vi "LINC Create Telemetry Definition.vi"(8 "error in (no error)":errorcluster, 10 "path":path, 11 "LINC session":refnum<class "LINC.lvclass">) -> (0 "error out":errorcluster, 3 "dup LINC session":refnum<class "LINC.lvclass">)   [LabVIEW 2018, in "STEPkgDriver_LINC.lvlib" / "LINC.lvclass"]
uses:
  LINC.lvclass
  STEPkgDriver_LINC.lvlib
  LINC Global Mode.ctl
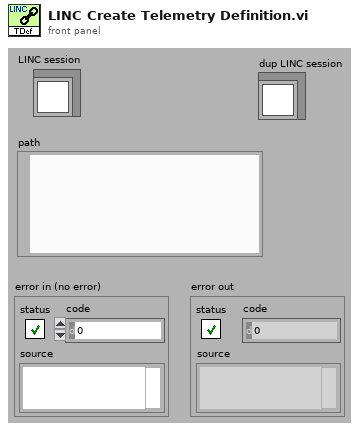
[diagram p1: front panel]
types:
  T1 = typedef "STEPkgDriver_LINC.lvlib/LINC Global Mode.ctl" = enum16{"INIT", "CLEAR", "ADD_PKT_HDR", "ADD_PKT", "GET_PKT_NAMES", "GET_PKT_DESC", "GET_PKT_HDR", "GET_PKT", "SET_PKT", "SET_DATA", "SIM_EN", "SIM_DS"}
  T2 = typedef "STEPkgDriver_LINC.lvlib/LINC Format Prototype.ctl" = cluster{"type":string, "bit offset":i32, "bit size":i32, "format":string, "unit":string, "description":string, "state values":i64[], "states":string[], "max":string, "min":string, "default":string, "array":bool, "bit element size":i32, "poly bound":dbl[], "poly scale":cluster{"coefficients":dbl[]}[], "labview size":i32, "simulate":bool, "ID":bool, "required":bool}
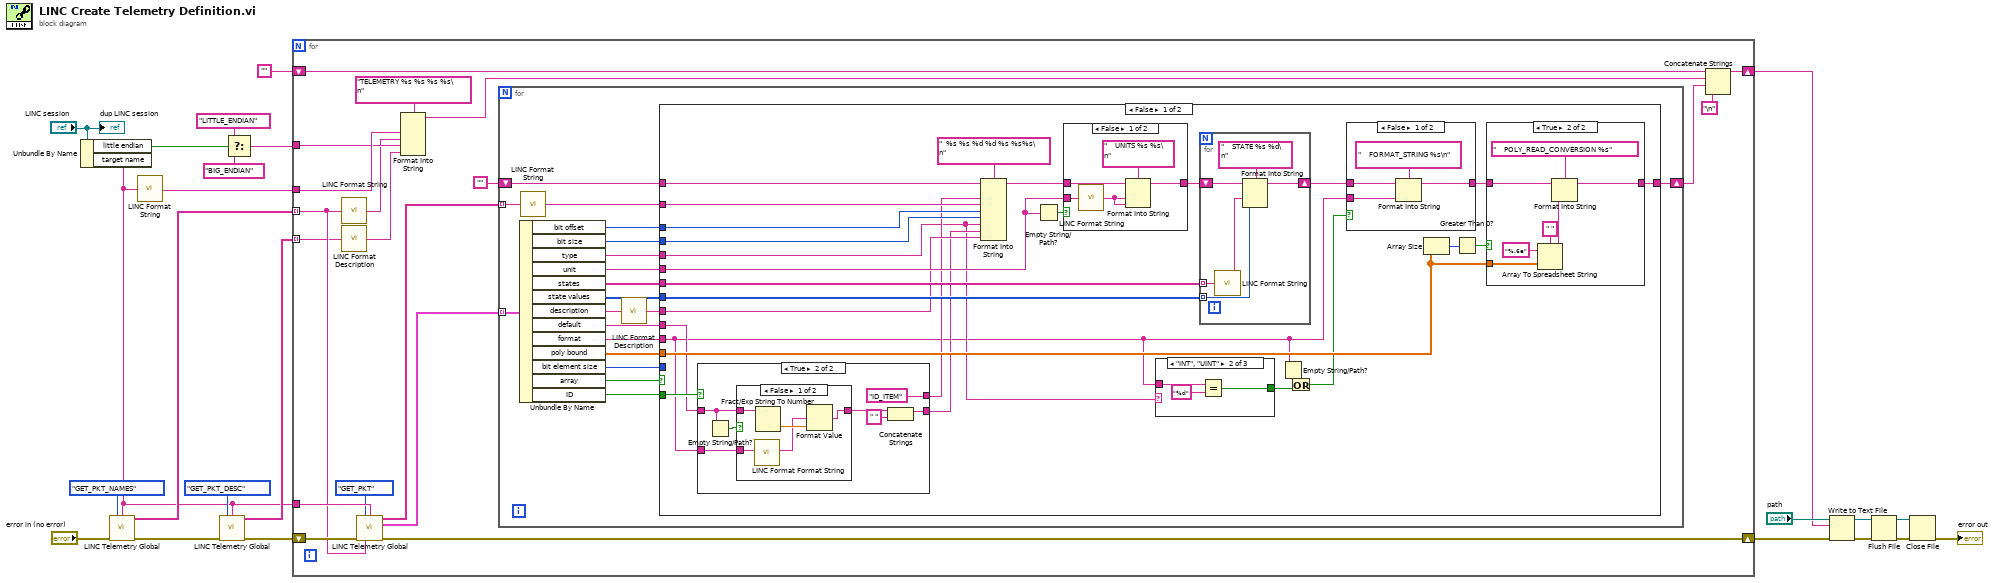
[diagram p0: block diagram]
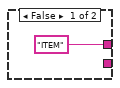
[diagram p2: hidden frame]
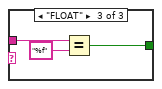
[diagram p5: hidden frame]
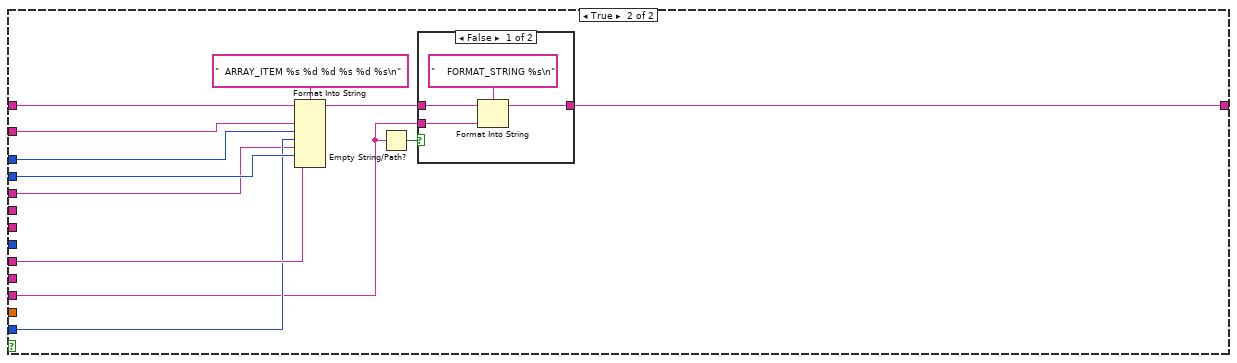
[diagram p9: hidden frame]
diagram:
  n1 = Unbundle By Name("LINC session") -> ("little endian"=w4:bool, "target name"=w1:string)
  n2 = call "LINC Telemetry Global.vi"("mode"=LINC_Global_Mode."GET_PKT_NAMES", "target name"=w1, "error in (no error)"="error in (no error)") -> ("values out"=w11:string[], "error out"=w15:errorcluster)  [unwired: 8 in, 3 out]
  n3 = call "LINC Format String.vi"("string in"=w1) -> ("string out"=w2:string)
  n4 = call "LINC Telemetry Global.vi"("mode"=LINC_Global_Mode."GET_PKT_DESC", "target name"=w1, "error in (no error)"=w15) -> ("values out"=w10:string[], "error out"=w14:errorcluster)  [unwired: 8 in, 3 out]
  n5 = Select(t="LITTLE_ENDIAN", s=w4, f="BIG_ENDIAN") -> (s? t:f=w3:string)
  n6 = for {
    tunnel: w2 -> [w42]
    shift-right: [w38] -> w16
    shift-left: "" -> [w39]
    shift-right: [w35] -> w12
    shift-left: w14 -> [w36]
    tunnel: w11 -> [w27] mode=indexing
    tunnel: w10 -> [w25] mode=indexing
    tunnel: w1 -> [w34]
    tunnel: w3 -> [w28]
    n7 = call "LINC Format String.vi"("string in"=w27) -> ("string out"=w26:string)
    n8 = call "LINC Format Description.vi"("string in"=w25) -> ("string out"=w24:string)
    n9 = call "LINC Telemetry Global.vi"("mode"=LINC_Global_Mode."GET_PKT", "target name"=w34, "error in (no error)"=w36, "packet name"=w27) -> ("values out"=w32:string[], "item formats out"=w33:T2[], "error out"=w35:errorcluster)  [unwired: 7 in, 2 out]
    n10 = Format Into String(format string="TELEMETRY %s %s %s %s\n", w42, w26, w28, w24) -> (resulting string=w31:string)  [unwired: 2 in, 1 out]
    n11 = for {
      shift-right: [w60] -> w30
      shift-left: "" -> [w61]
      tunnel: w32 -> [w48] mode=indexing
      tunnel: w33 -> [w56] mode=indexing
      n12 = Unbundle By Name(w56) -> ("bit offset"=w55:i32, "bit size"=w53:i32, "type"=w59:string, "unit"=w58:string, "states"=w57:string[], "state values"=w54:i64[], "description"=w46:string, "default"=w43:string, "format"=w49:string, "poly bound"=w51:dbl[], "bit element size"=w44:i32, "array"=w52:bool, "ID"=w50:bool)
      n13 = call "LINC Format String.vi"("string in"=w48) -> ("string out"=w47:string)
      n14 = call "LINC Format Description.vi"("string in"=w46) -> ("string out"=w45:string)
      n15 = case shown="False" w52 {
        tunnel: w61 -> [w87 w144]
        tunnel: [w73 w137] -> w60
        tunnel: w45 -> [w68 w141]
        tunnel: w59 -> [w64 w136]
        tunnel: w49 -> [w62 w135]
        tunnel: w58 -> [w82 _]
        tunnel: w57 -> [w81 _]
        tunnel: w47 -> [w80 w143]
        tunnel: w55 -> [w79 w142]
        tunnel: w54 -> [w78 _]
        tunnel: w53 -> [w77 w140]
        tunnel: w44 -> [_ w139]
        tunnel: w51 -> [w72 _]
        tunnel: w50 -> [w67 _]
        tunnel: w43 -> [w63 _]
        frame False {
          n16 = case shown="True" w67 {
            tunnel: ["ITEM" "ID_ITEM"] -> w66
            tunnel: w63 -> [_ w92]
            tunnel: [_ w94] -> w65
            tunnel: w62 -> [_ w90]
            frame False {
            }
            frame True {
              n17 = Empty String/Path?(string/path=w92) -> (empty?=w93:bool)
              n18 = case shown="False" w93 {
                tunnel: w90 -> [w101 _]
                tunnel: w92 -> [w100 w102]
                tunnel: [w97 w102] -> w91
                frame False {
                  n19 = call "LINC Format Format String.vi"("format in"=w101) -> ("format out"=w98:string)  [unwired: 10 in]
                  n20 = Fract/Exp String To Number(string=w100) -> (number=w99:dbl)  [unwired: 3 in, 1 out]
                  n21 = Format Value(format string=w98, value (0)=w99) -> (output string=w97:string)  [unwired: 1 in]
                }
                frame True {
                }
              }
              n22 = Concatenate Strings(w91, " " ("string")) -> (w94:string)
            }
          }
          n23 = Format Into String(format string="  %s %s %d %d %s %s%s\n", initial string=w87, w66, w80, w79, w77, w64, w65, w68) -> (resulting string=w84:string)  [unwired: 1 in, 1 out]
          n24 = Empty String/Path?(string/path=w82) -> (empty?=w85:bool)
          n25 = case shown="False" w85 {
            tunnel: w84 -> [w120 w122]
            tunnel: [w119 w122] -> w83
            tunnel: w82 -> [w118 _]
            frame False {
              n26 = call "LINC Format String.vi"("string in"=w118) -> ("string out"=w117:string)
              n27 = Format Into String(format string="    UNITS %s %s\n", initial string=w120, w117, w117) -> (resulting string=w119:string)  [unwired: 1 in, 1 out]
            }
            frame True {
            }
          }
          n28 = case shown="\"INT\", \"UINT\"" w64 {
            tunnel: w62 -> [_ w104 w107]
            tunnel: [_ w103 w106] -> w69
            frame Default {
            }
            frame "INT", "UINT" {
              n29 = Equal?(x=w104, y="%d") -> (x = y?=w103:bool)
            }
            frame "FLOAT" {
              n30 = Equal?(x=w107, y="%f") -> (x = y?=w106:bool)
            }
          }
          n31 = for {
            shift-right: [w132] -> w86
            shift-left: w83 -> [w133]
            tunnel: w81 -> [w129] mode=indexing
            tunnel: w78 -> [w130] mode=indexing
            n32 = call "LINC Format String.vi"("string in"=w129) -> ("string out"=w128:string)
            n33 = Format Into String(format string="    STATE %s %d\n", initial string=w133, w128, w130) -> (resulting string=w132:string)  [unwired: 1 in, 1 out]
          }
          n34 = Empty String/Path?(string/path=w62) -> (empty?=w71:bool)
          n35 = Or(x=w71, y=w69) -> (x .or. y?=w70:bool)
          n36 = case shown="False" w70 {
            tunnel: w86 -> [w125 w127]
            tunnel: [w124 w127] -> w74
            tunnel: w62 -> [w123 _]
            frame False {
              n37 = Format Into String(format string="    FORMAT_STRING %s\n", initial string=w125, w123) -> (resulting string=w124:string)  [unwired: 1 in, 1 out]
            }
            frame True {
            }
          }
          n38 = Array Size(array=w72) -> (size(s)=w76:i32)
          n39 = Greater Than 0?(x=w76) -> (x > 0?=w75:bool)
          n40 = case shown="True" w75 {
            tunnel: w74 -> [w109 w115]
            tunnel: [w109 w114] -> w73
            tunnel: w72 -> [_ w111]
            frame False {
            }
            frame True {
              n41 = Array To Spreadsheet String(delimiter (Tab)=" ", array=w111, 3:"%.6e" ("format string")) -> (spreadsheet string=w110:string)
              n42 = Format Into String(format string="    POLY_READ_CONVERSION %s", initial string=w115, w110) -> (resulting string=w114:string)  [unwired: 1 in, 1 out]
            }
          }
        }
        frame True {
          n43 = Format Into String(format string="  ARRAY_ITEM %s %d %d %s %d %s\n", initial string=w144, w143, w142, w139, w136, w140, w141) -> (resulting string=w138:string)  [unwired: 1 in, 1 out]
          n44 = Empty String/Path?(string/path=w135) -> (empty?=w134:bool)
          n45 = case shown="False" w134 {
            tunnel: w138 -> [w148 w150]
            tunnel: [w147 w150] -> w137
            tunnel: w135 -> [w146 _]
            frame False {
              n46 = Format Into String(format string="    FORMAT_STRING %s\n", initial string=w148, w146) -> (resulting string=w147:string)  [unwired: 1 in, 1 out]
            }
            frame True {
            }
          }
        }
      }
    }
    n47 = Concatenate Strings(w39, w31, w30, "\n") -> (w38:string)
  }
  n48 = Write to Text File(file (use dialog)="path", text=w16, error in=w12) -> (refnum out=w21:refnum<file>, error out=w22:errorcluster)  [unwired: 2 out]
  n49 = Flush File(refnum=w21, error in=w22) -> (refnum out=w19:refnum<file>, error out=w20:errorcluster)
  n50 = Close File(refnum=w19, error in=w20) -> (error out=→"error out":errorcluster)  [unwired: 1 out]
  "dup LINC session" <- "LINC session"
